vi "Main.vi"() -> ()   [LabVIEW 2020, in "ZLG_CAN.lvlib"]
doc: "This template is based off of the Queued Message Handler design pattern and the Queued Message Handler project template that ships with LabVIEW.\n\nThe main difference is that the queue is private to this module and communication between modules is performed via Broadcast and Request events.\n\nRequest events are wrapped in public API methods and are handled in the Event Handling Loop (EHL) of this VI. Any module can register for Broadcast events sent by this module. The EHL generates messages based on user interface actions.\n\nThe Message Handling Loop (MHL) processes messages generated by the EHL, or by other messages. The messages are string values, so new messages can be added easily to the Message Cases case structure in the MHL. Each message cluster can also provide an optional value for Message Data, which is a variant that can be converted to whatever message-specific data is required.\n_____\nBased on Delacor QMH Project Template 4.1.0.59."
uses:
  ZLG_CAN.lvlib
  <vilib>/Delacor/Delacor QMH/Libraries/Module Admin_class/Delacor_lib_QMH_Module Admin.lvclass
  CAN_OBJ_R.ctl
  Module Data--cluster.ctl
  <vilib>/Delacor/Delacor QMH/Libraries/Message Queue_class/Delacor_lib_QMH_Message Queue.lvclass/Delacor_lib_QMH_Message Queue.ctl
  Stop Argument--cluster.ctl
  <vilib>/Delacor/Delacor QMH/Libraries/Module Admin_class/Delacor_lib_QMH_Module Admin.lvclass/Delacor_lib_QMH_Module Admin.ctl
  Open_CAN Argument--cluster.ctl
  Init_CAN Argument--cluster.ctl
  Start_CAN Argument--cluster.ctl
  Start_CAN (Reply Payload)--cluster.ctl
  Sent_CAN Argument--cluster.ctl
  CAN_Frame.ctl
  Close_CAN Argument--cluster.ctl
  Reset_CAN Argument--cluster.ctl
  Recive_CAN Argument--cluster.ctl
  Recive_Wait Argument--cluster.ctl
  Recive_Wait (Reply Payload)--cluster.ctl
  Sent_Recive Argument--cluster.ctl
  Sent_Recive (Reply Payload)--cluster.ctl
  <vilib>/Utility/miscctls.llb/LVPointTypeDef.ctl
  CAN_OBJ_T.ctl
  <vilib>/Delacor/Delacor QMH/Libraries/Message Queue_class/Delacor_lib_QMH_Enqueue Message (Single).vi
  <vilib>/Delacor/Delacor QMH/Libraries/Module Admin_class/Delacor_lib_QMH_Get External Launch.vi
  <vilib>/Utility/error.llb/Error Cluster From Error Code.vi
  <vilib>/ErrorRing/Error Ring.xnode
  <vilib>/Delacor/Delacor QMH/Libraries/Message Queue_class/Delacor_lib_QMH_Message Queue.lvclass
  ControlCAN.dll
panel:
  out "CAN_OBJ_RN":T1[](array[typedef])
  out "CAN 通道":u32
  out "索引":u32
  out "设备类型":u32
  in  "Simulate MHL Error":bool
  in  "Simulate EHL Error":bool
  out "error out":errorcluster
  in  "Module Admin":refnum<class "Delacor_lib_QMH_Module Admin.lvclass">
  out "Status":string
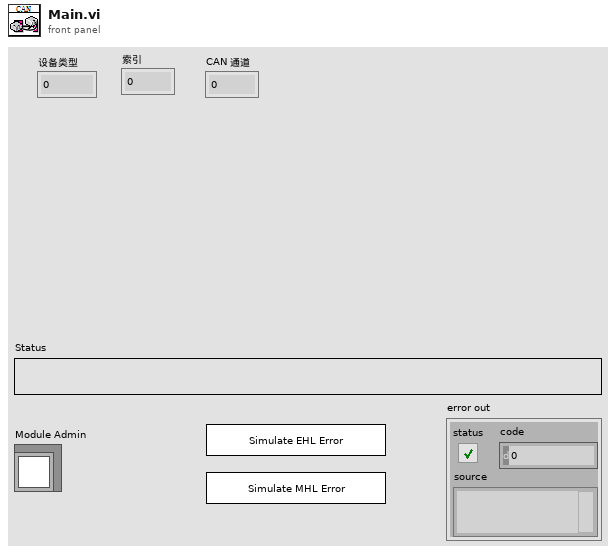
[diagram p1: front panel]
types:
  T1 = typedef "ZLG_CAN.lvlib/CAN_OBJ_R.ctl" = cluster{"ID":u32, "TimeStamp":u32, "TimeFlag":u8, "SendType":u8, "RemoteFlag":u8, "ExternFlag":u8, "DataLen":u8, "数值":u8, "数值":u8, "数值":u8, "数值":u8, "数值":u8, "数值":u8, "数值":u8, "数值":u8, "数值":u8, "数值":u8, "数值":u8}
  T2 = typedef "ZLG_CAN.lvlib/Request Events--cluster.ctl" = cluster{"Stop Module":refnum<user-event>, "Show Panel":refnum<user-event>, "Hide Panel":refnum<user-event>, "Get Module Execution Status":refnum<user-event>, "Show Diagram":refnum<user-event>, "Open_CAN":refnum<user-event>, "Init_CAN":refnum<user-event>, "Start_CAN":refnum<user-event>, "Sent_CAN":refnum<user-event>, "Close_CAN":refnum<user-event>, "Reset_CAN":refnum<user-event>, "Recive_CAN":refnum<user-event>, "Recive_Wait":refnum<user-event>, "Sent_Recive":refnum<user-event>}
  T3 = typedef "ZLG_CAN.lvlib/Module Data--cluster.ctl" = cluster{"Status":string}
  T4 = enum32{"invalid lock state", "Not Locked", "Locked (No Password)", "Password-protected"}
  T5 = typedef "ZLG_CAN.lvlib/Stop Argument--cluster.ctl" = cluster{"Origin":string, "Exit via Stop Module Req?":bool, "Wait for Module to stop?":bool}
  T6 = typedef "ZLG_CAN.lvlib/Open_CAN Argument--cluster.ctl" = cluster{"设备类型":u32, "索引":u32, "CAN 通道":u32}
  T7 = typedef "ZLG_CAN.lvlib/Init_CAN Argument--cluster.ctl" = cluster{"波特率":u32}
  T8 = typedef "ZLG_CAN.lvlib/Start_CAN Argument--cluster.ctl" = cluster{"布尔":bool, "Wait Notifier":refnum<notifier>, "wait for reply":bool}
  T9 = typedef "ZLG_CAN.lvlib/Sent_CAN Argument--cluster.ctl" = cluster{"ID":u32, "帧类型":u8, "帧格式":u8, "帧长度":u8, "CAN_FRAME":T10}
  T10 = typedef "ZLG_CAN.lvlib/CAN_Frame.ctl" = cluster{"[0]":u8, "[1]":u8, "[2]":u8, "[3]":u8, "[4]":u8, "[5]":u8, "[6]":u8, "[7]":u8}
  T11 = typedef "ZLG_CAN.lvlib/Close_CAN Argument--cluster.ctl" = cluster{"设备类型":u32, "索引":u32}
  T12 = typedef "ZLG_CAN.lvlib/Reset_CAN Argument--cluster.ctl" = cluster{"设备类型":u32, "索引":u32, "CAN 通道":u32}
  T13 = typedef "ZLG_CAN.lvlib/Recive_CAN Argument--cluster.ctl" = cluster{"布尔":bool}
  T14 = typedef "ZLG_CAN.lvlib/Recive_Wait Argument--cluster.ctl" = cluster{"Wait Notifier":refnum<notifier>, "wait for reply":bool}
  T15 = typedef "ZLG_CAN.lvlib/Sent_Recive Argument--cluster.ctl" = cluster{"ID":u32, "帧类型":u8, "帧格式":u8, "CAN_FRAME":T10, "帧长度":u8, "Wait Notifier":refnum<notifier>, "wait for reply":bool}
  T16 = typedef "LVPointTypeDef.ctl" = cluster{"Horizontal":i16, "Vertical":i16}
  T17 = enum32{"Invalid", "Standard", "Closed", "Hidden", "Minimized", "Maximized"}
  T18 = cluster{"AccCode":u32, "AccMask":u32, "Reserved":u32, "Filter":u8, "Timing0":u8, "Timing1":u8, "Mode":u8}
  T19 = typedef "ZLG_CAN.lvlib/CAN_OBJ_T.ctl" = cluster{"ID":u32, "TimeStamp":u32, "TimeFlag":u8, "SendType":u8, "RemoteFlag":u8, "ExternFlag":u8, "DataLen":u8, "CAN_Bit_0":u8, "CAN_Bit_1":u8, "CAN_Bit_2":u8, "CAN_Bit_3":u8, "CAN_Bit_4":u8, "CAN_Bit_5":u8, "CAN_Bit_6":u8, "CAN_Bit_7":u8, "CAN_Bit_8":u8, "CAN_Bit_9":u8, "CAN_Bit_10":u8}
  T20 = typedef "ZLG_CAN.lvlib/Start_CAN (Reply Payload)--cluster.ctl" = cluster{"Success":bool, "Start_CAN_error":errorcluster}
  T21 = typedef "ZLG_CAN.lvlib/Recive_Wait (Reply Payload)--cluster.ctl" = cluster{"Can_Receive":T1[], "Recive_Wait_error":errorcluster}
  T22 = typedef "ZLG_CAN.lvlib/Sent_Recive (Reply Payload)--cluster.ctl" = cluster{"Receive":T1[], "Sent_Recive_error":errorcluster}
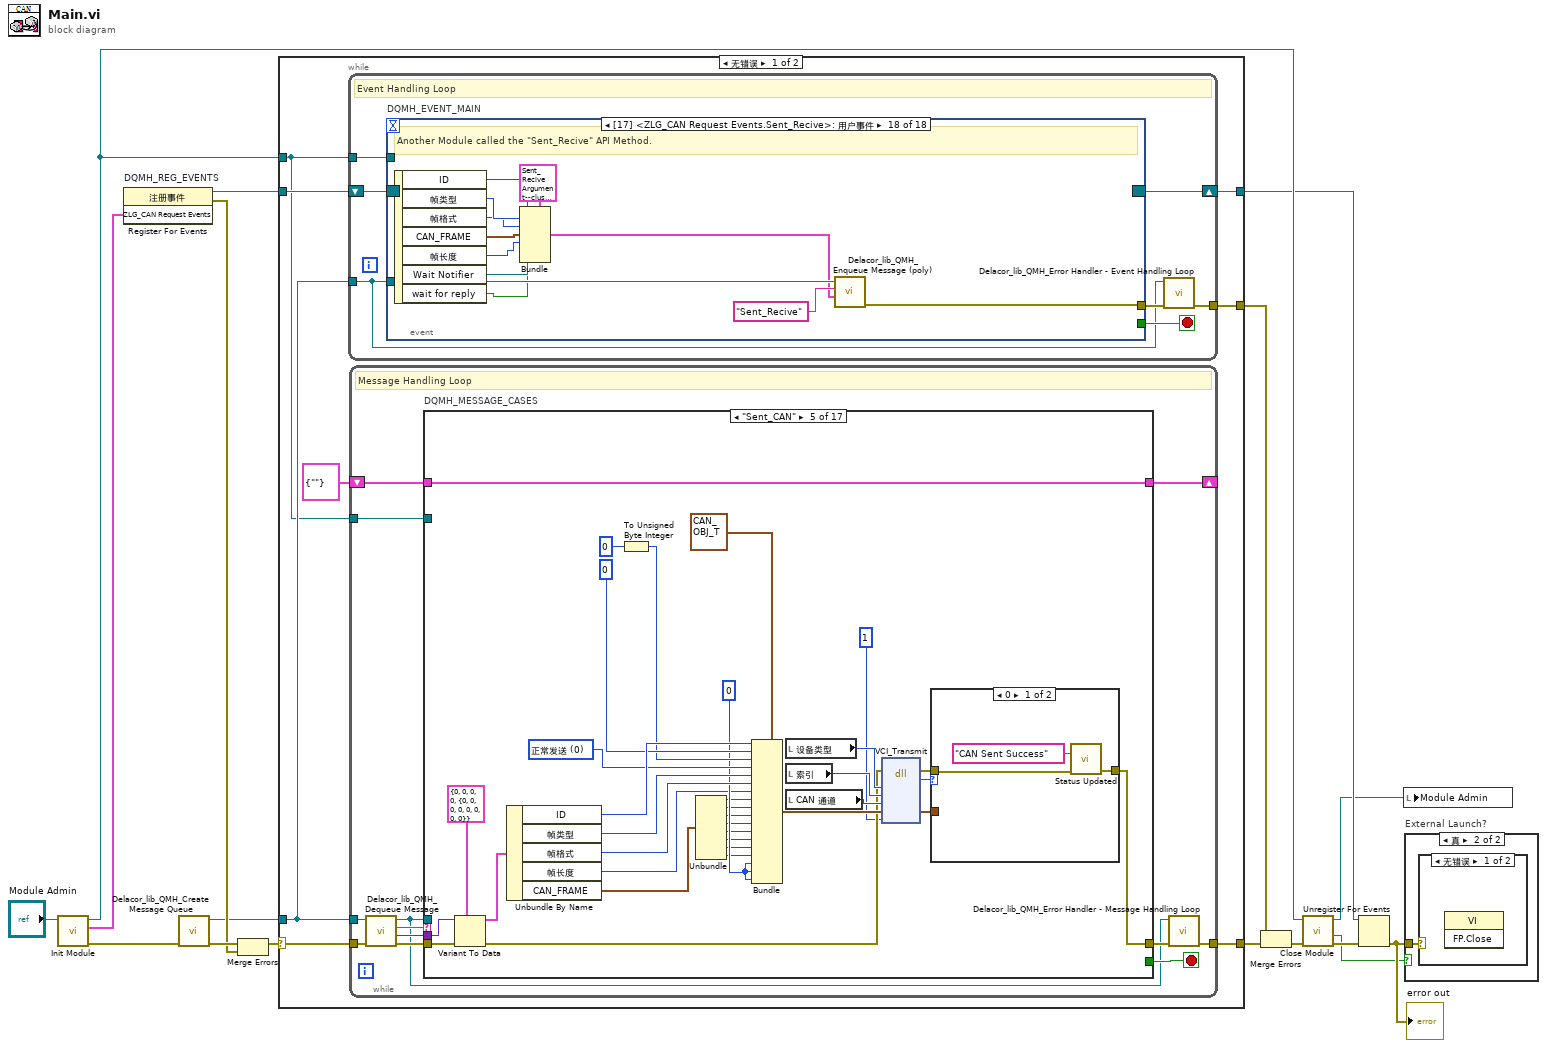
[diagram p0: block diagram]
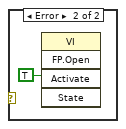
[diagram p3: hidden frame]
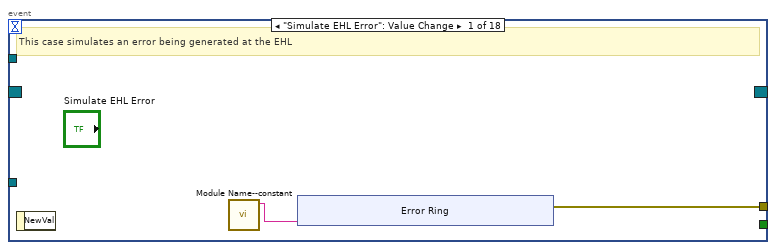
[diagram p4: hidden frame]
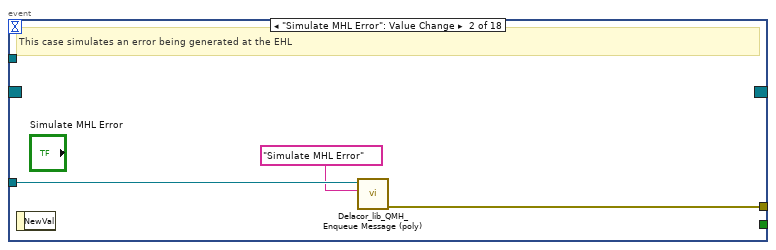
[diagram p5: hidden frame]
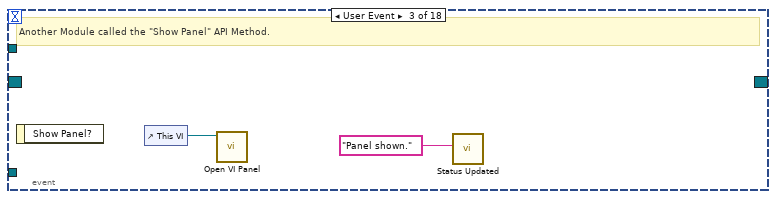
[diagram p6: hidden frame]
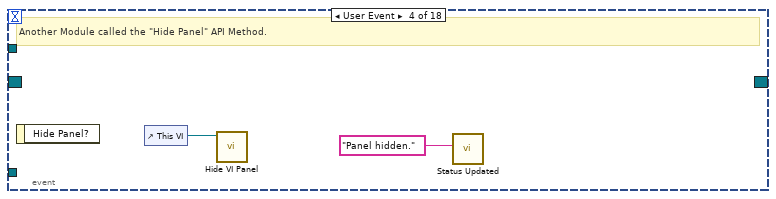
[diagram p7: hidden frame]
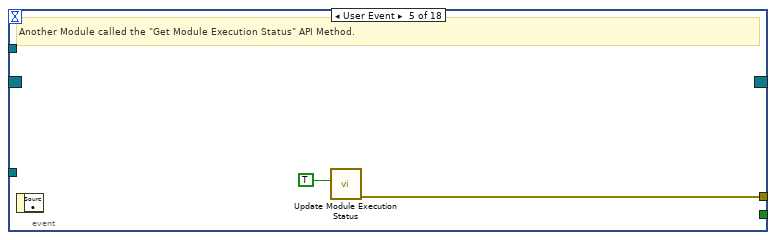
[diagram p8: hidden frame]
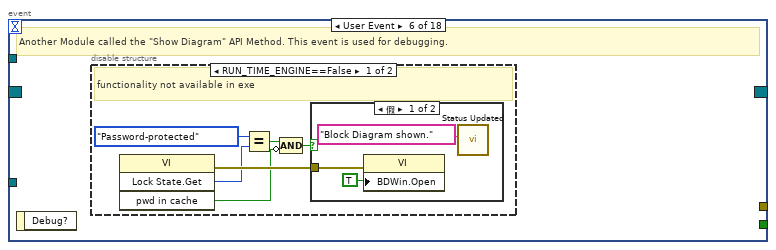
[diagram p9: hidden frame]
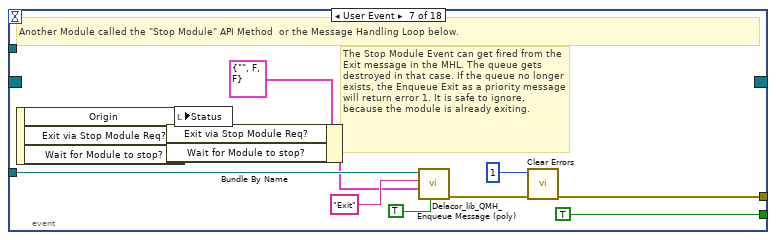
[diagram p12: hidden frame]
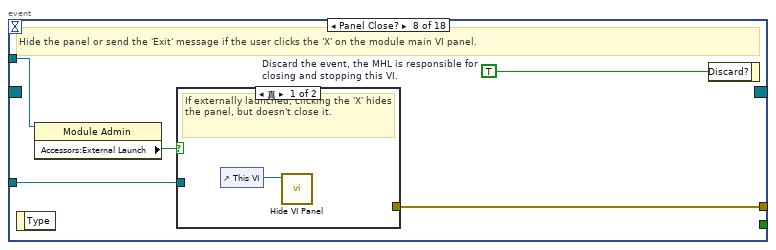
[diagram p13: hidden frame]
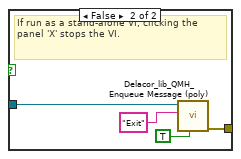
[diagram p14: hidden frame]
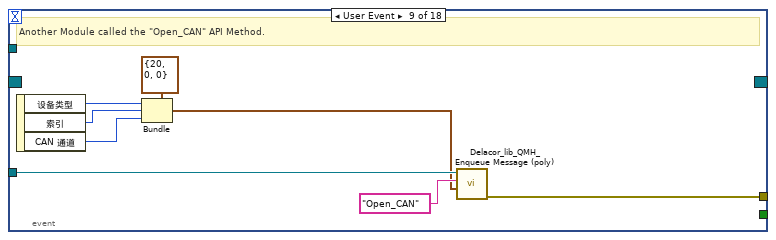
[diagram p15: hidden frame]
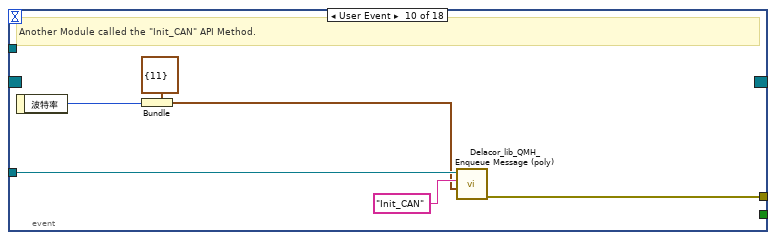
[diagram p16: hidden frame]
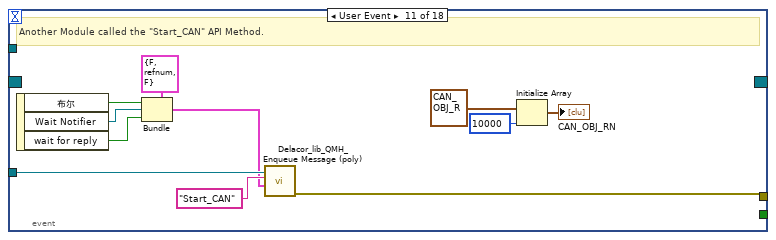
[diagram p17: hidden frame]
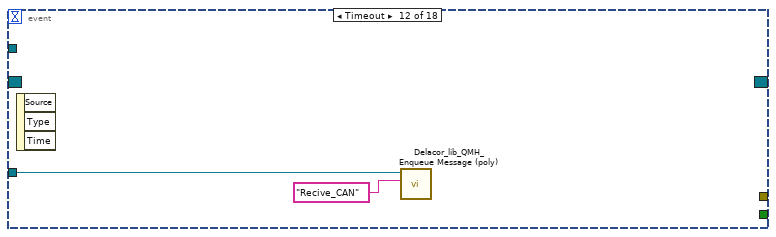
[diagram p18: hidden frame]
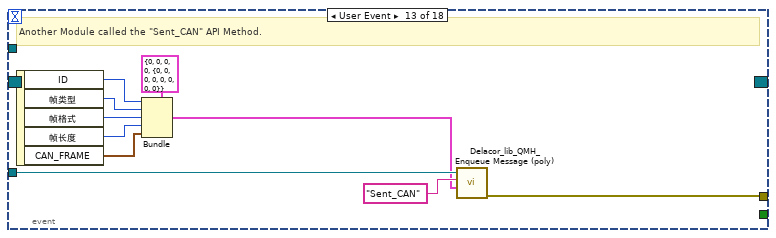
[diagram p19: hidden frame]
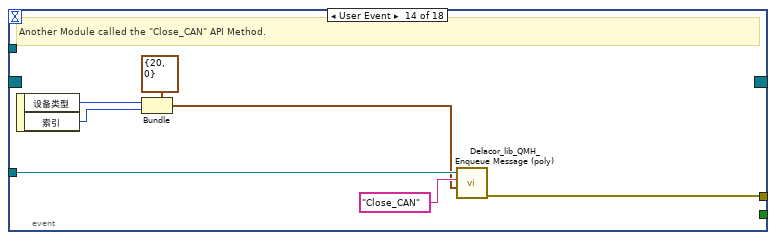
[diagram p20: hidden frame]
diagram:
  n1 = call "Init Module.vi"("Singleton Module Admin in"="Module Admin") -> ("error out"=w16:errorcluster, "ZLG_CAN Request Events"=w5:T2, "Singleton Module Admin out"=w8:refnum<class "Delacor_lib_QMH_Module Admin.lvclass">)  [unwired: 8 in]
  n2 = register-events "DQMH_REG_EVENTS"(w5) -> (reference out=w6:refnum<event-registration>, error out=w9:errorcluster)  [unwired: 2 in]
  n3 = call <vilib>:"Delacor_lib_QMH_Create Message Queue.vi"("error in"=w16) -> ("error out"=w11:errorcluster, "Message Queue"=w4:refnum<class "Delacor_lib_QMH_Message Queue.lvclass">)  [unwired: 9 in]
  n4 = Merge Errors(w11, w9) -> (w10:errorcluster)
  n5 = case shown="无错误" w10 {
    selector: w10 -> [w23 w581]
    tunnel: [w25 w581] -> w17
    tunnel: [w22 w578] -> w7
    tunnel: w6 -> [w20 w578]
    tunnel: w4 -> [w19 _]
    tunnel: [w24 _] -> w14
    tunnel: w8 -> [w18 w574]
    frame No Error {
      n6 = while {
        tunnel: w19 -> [w26]
        shift-right: [w29] -> w22
        shift-left: w20 -> [w30]
        tunnel: [w31] -> w24
        tunnel: w18 -> [w27]
        stop <- w28 stop-if-true
        # "Event Handling Loop"
        n7 = event "DQMH_EVENT_MAIN" shown="[17] <ZLG_CAN Request Events.Sent_Recive>: 用户事件" {
          selector: w30 -> [_ _ _ _ _ _ _ _ _ _ _ _ _ _ _ _ _ _]
          dyn-events: [_ _ _ _ _ _ _ _ _ _ _ _ _ _ _ _ _ _] -> w29
          timeout: _ -> [_ _ _ _ _ _ _ _ _ _ _ _ _ _ _ _ _ _]
          tunnel: [_ _ _ _ _ _ TRUE ("Discard?") _ _ _ _ _ _ _ _ _ _ _] -> w28
          tunnel: w26 -> [_ w43 _ _ _ _ w67 w74 w89 w95 w106 w107 w118 w125 w133 w139 w146 w158]
          tunnel: [w34 w44 _ _ w50 _ w70 w76 w82 w90 w101 _ w113 w119 w128 w134 w140 w147] -> w32
          tunnel: w27 -> [_ _ _ _ _ _ _ w73 _ _ _ _ _ _ _ _ _ _]
          event "Simulate EHL Error": Value Change {
            # "This case simulates an error being generated at the EHL"
            n8 = event-data() -> ()  [unwired: 1 in, 1 out]
            n9 = call "Module Name--constant.vi"() -> ("Module Name"=w33:string)  [unwired: 11 in]
            n10 = xnode "Error Ring"("参数 0"=w33) -> ("错误输出"=w34:errorcluster)
          }
          event "Simulate MHL Error": Value Change {
            # "This case simulates an error being generated at the EHL"
            n11 = event-data() -> ()  [unwired: 1 in, 1 out]
            n12 = call-poly <vilib>:"Delacor_lib_QMH_Enqueue Message (poly).vi"("Message"="Simulate MHL Error", "Message Queue in"=w43) -> ("error out"=w44:errorcluster)  [unwired: 8 in, 1 out]
          }
          event User Event {
            # "Another Module called the \"Show Panel\" API Method."
            n13 = event-data() -> ()  [unwired: 1 in, 1 out]
            n14 = control-ref of="This VI"() -> (w46:refnum<vi>)
            n15 = call "Open VI Panel.vi"("VI"=w46) -> ()  [unwired: 10 in, 1 out]
            n16 = call "Status Updated.vi"("Status"="Panel shown." ("format string")) -> ()  [unwired: 10 in, 1 out]
          }
          event User Event {
            # "Another Module called the \"Hide Panel\" API Method."
            n17 = event-data() -> ()  [unwired: 1 in, 1 out]
            n18 = control-ref of="This VI"() -> (w48:refnum<vi>)
            n19 = call "Hide VI Panel.vi"("VI"=w48) -> ()  [unwired: 10 in, 1 out]
            n20 = call "Status Updated.vi"("Status"="Panel hidden." ("format string")) -> ()  [unwired: 10 in, 1 out]
          }
          event User Event {
            # "Another Module called the \"Get Module Execution Status\" API Method."
            n21 = event-data() -> ()  [unwired: 1 in, 1 out]
            n22 = call "Update Module Execution Status.vi"("Running?"=TRUE) -> ("error out"=w50:errorcluster)  [unwired: 10 in]
          }
          event User Event {
            # "Another Module called the \"Show Diagram\" API Method. This event is used for debugging."
            n23 = event-data() -> ()  [unwired: 1 in, 1 out]
            n24 = disable-structure shown="RUN_TIME_ENGINE==False" {
              frame condition #0 (active) {
                # "functionality not available in exe"
                n25 = invoke class="VI" method="Lock State.Get"() -> (error out=w56:errorcluster, "Get Lock State"=w55:T4, "pwd in cache"=w52:bool)  [unwired: 4 in, 1 out]
                n26 = Equal?(x=T4."Password-protected", y=w55) -> (x = y?=w53:bool)
                n27 = Compound Arithmetic op=AND(w53, invert w52) -> (w51:bool)
                n28 = case "条件结构" shown="假" w51 {
                  tunnel: w56 -> [w59 _]
                  frame False {
                    n29 = property class="VI"(error in=w59, "BDWin.Open"=TRUE ("Block Diagram Window:Open")) -> ()  [unwired: 1 in, 2 out]
                    n30 = call "Status Updated.vi"("Status"="Block Diagram shown." ("format string")) -> ()  [unwired: 10 in, 1 out]
                  }
                  frame True {
                    # "Password-protected VI, and the password is not in the cache. Do not show the diagram."
                  }
                }
              }
              frame condition #1 {
              }
            }
          }
          event User Event {
            # "The Stop Module Event can get fired from the Exit message in the MHL. The queue gets destroyed in that case. If the queue no longer exists, the Enqueue Exit as a priority message will return error 1. It is safe to ignore, because the module is already exiting."
            # "Another Module called the \"Stop Module\" API Method  or the Message Handling Loop below."
            n31 = event-data() -> ("Origin"=w66:string, "Exit via Stop Module Req?"=w62:bool, "Wait for Module to stop?"=w61:bool)  [unwired: 1 in]
            n32 = Bundle By Name(cluster=T5 {"Origin"="", "Exit via Stop Module Req?"=FALSE, "Wait for Module to stop?"=FALSE} ("Stop Argument"), "Exit via Stop Module Req?"=w62, "Wait for Module to stop?"=w61) -> (w60:T5)
            n33 = local write "Status"(w66) -> ()
            n34 = call-poly <vilib>:"Delacor_lib_QMH_Enqueue Message (poly).vi"("Priority Message? (F)"=TRUE, "Message Data"=w60, "Message"="Exit", "Message Queue in"=w67) -> ("error out"=w71:errorcluster)  [unwired: 6 in, 1 out]
            n35 = call <vilib>:"Clear Errors.vi"("error in (no error)"=w71, "specific error code to clear (0: all)"=1) -> ("error out"=w70:errorcluster)  [unwired: 4 in, 1 out]
          }
          event Panel Close? {
            w75 = TRUE  # Discard the event, the MHL is responsible for closing and stopping this VI.
            # "Hide the panel or send the 'Exit' message if the user clicks the 'X' on the module main VI panel."
            n36 = event-data() -> ()  [unwired: 1 in, 1 out]
            n37 = property class="Module Admin"(reference=w73) -> ("Accessors:External Launch"=w72:bool)  [unwired: 1 in, 2 out]
            n38 = case "条件结构" shown="真" w72 {
              tunnel: w74 -> [_ w80]
              tunnel: [_ w81] -> w76
              frame True {
                # "If externally launched, clicking the 'X' hides the panel, but doesn't close it."
                n39 = control-ref of="This VI"() -> (w77:refnum<vi>)
                n40 = call "Hide VI Panel.vi"("VI"=w77) -> ()  [unwired: 10 in, 1 out]
              }
              frame False {
                # "If run as a stand-alone VI, clicking the panel 'X' stops the VI."
                n41 = call-poly <vilib>:"Delacor_lib_QMH_Enqueue Message (poly).vi"("Priority Message? (F)"=TRUE, "Message"="Exit", "Message Queue in"=w80) -> ("error out"=w81:errorcluster)  [unwired: 7 in, 1 out]
              }
            }
            n42 = event-data("Discard?"=w75) -> ()  [unwired: 1 in, 1 out]
          }
          event User Event {
            # "Another Module called the \"Open_CAN\" API Method."
            n43 = event-data() -> ("设备类型"=w85:u32, "索引"=w84:u32, "CAN 通道"=w83:u32)  [unwired: 1 in]
            n44 = Bundle(cluster=T6 {"设备类型"=20, "索引"=0, "CAN 通道"=0} ("Open_CAN Argument"), "设备类型"=w85, "索引"=w84, "CAN 通道"=w83) -> (w86:T6)
            n45 = call-poly <vilib>:"Delacor_lib_QMH_Enqueue Message (poly).vi"("Message Data"=w86, "Message"="Open_CAN", "Message Queue in"=w89) -> ("error out"=w82:errorcluster)  [unwired: 7 in, 1 out]
          }
          event User Event {
            # "Another Module called the \"Init_CAN\" API Method."
            n46 = event-data() -> ("波特率"=w91:u32)  [unwired: 1 in]
            n47 = Bundle(cluster=T7 {"波特率"=11} ("Init_CAN Argument"), "波特率"=w91) -> (w92:T7)
            n48 = call-poly <vilib>:"Delacor_lib_QMH_Enqueue Message (poly).vi"("Message Data"=w92, "Message"="Init_CAN", "Message Queue in"=w95) -> ("error out"=w90:errorcluster)  [unwired: 7 in, 1 out]
          }
          event User Event {
            # "Another Module called the \"Start_CAN\" API Method."
            n49 = event-data() -> ("布尔"=w102:bool, "Wait Notifier"=w100:refnum<notifier>, "wait for reply"=w99:bool)  [unwired: 1 in]
            n50 = Bundle(cluster=T8 {"布尔"=FALSE, "Wait Notifier"=refnum, "wait for reply"=FALSE} ("Start_CAN Argument"), "布尔"=w102, "Wait Notifier"=w100, "wait for reply"=w99) -> (w103:T8)
            n51 = call-poly <vilib>:"Delacor_lib_QMH_Enqueue Message (poly).vi"("Message Data"=w103, "Message"="Start_CAN", "Message Queue in"=w106) -> ("error out"=w101:errorcluster)  [unwired: 7 in, 1 out]
            n52 = Initialize Array(T1 {"ID"=0, "TimeStamp"=0, "TimeFlag"=0, "SendType"=1, "RemoteFlag"=0, "ExternFlag"=0, "DataLen"=8, "数值"=0, "数值"=0, "数值"=0, "数值"=0, "数值"=0, "数值"=0, "数值"=0, "数值"=0, "数值"=0, "数值"=0, "数值"=0} ("CAN_OBJ_R"), 10000 ("维数大小")) -> (→"CAN_OBJ_RN":T1[])
          }
          event Timeout {
            n53 = event-data() -> ()  [unwired: 1 in, 3 out]
            n54 = call-poly <vilib>:"Delacor_lib_QMH_Enqueue Message (poly).vi"("Message"="Recive_CAN", "Message Queue in"=w107) -> ()  [unwired: 8 in, 2 out]
          }
          event User Event {
            # "Another Module called the \"Sent_CAN\" API Method."
            n55 = event-data() -> ("ID"=w114:u32, "帧类型"=w112:u8, "帧格式"=w111:u8, "帧长度"=w110:u8, "CAN_FRAME"=w109:T10)  [unwired: 1 in]
            n56 = Bundle(cluster=T9 {"ID"=0, "帧类型"=0, "帧格式"=0, "帧长度"=0, "CAN_FRAME"={"[0]"=0, "[1]"=0, "[2]"=0, "[3]"=0, "[4]"=0, "[5]"=0, "[6]"=0, "[7]"=0}} ("Sent_CAN Argument"), "ID"=w114, "帧类型"=w112, "帧格式"=w111, "帧长度"=w110, "CAN_FRAME"=w109) -> (w115:T9)
            n57 = call-poly <vilib>:"Delacor_lib_QMH_Enqueue Message (poly).vi"("Message Data"=w115, "Message"="Sent_CAN", "Message Queue in"=w118) -> ("error out"=w113:errorcluster)  [unwired: 7 in, 1 out]
          }
          event User Event {
            # "Another Module called the \"Close_CAN\" API Method."
            n58 = event-data() -> ("设备类型"=w121:u32, "索引"=w120:u32)  [unwired: 1 in]
            n59 = Bundle(cluster=T11 {"设备类型"=20, "索引"=0} ("Close_CAN Argument"), "设备类型"=w121, "索引"=w120) -> (w122:T11)
            n60 = call-poly <vilib>:"Delacor_lib_QMH_Enqueue Message (poly).vi"("Message Data"=w122, "Message"="Close_CAN", "Message Queue in"=w125) -> ("error out"=w119:errorcluster)  [unwired: 7 in, 1 out]
          }
          event User Event {
            # "Another Module called the \"Reset_CAN\" API Method."
            n61 = event-data() -> ("设备类型"=w129:u32, "索引"=w127:u32, "CAN 通道"=w126:u32)  [unwired: 1 in]
            n62 = Bundle(cluster=T12 {"设备类型"=20, "索引"=0, "CAN 通道"=0} ("Reset_CAN Argument"), "设备类型"=w129, "索引"=w127, "CAN 通道"=w126) -> (w130:T12)
            n63 = call-poly <vilib>:"Delacor_lib_QMH_Enqueue Message (poly).vi"("Message Data"=w130, "Message"="Reset_CAN", "Message Queue in"=w133) -> ("error out"=w128:errorcluster)  [unwired: 7 in, 1 out]
          }
          event User Event {
            # "Another Module called the \"Recive_CAN\" API Method."
            n64 = event-data() -> ("布尔"=w135:bool)  [unwired: 1 in]
            n65 = Bundle(cluster=T13 {"布尔"=FALSE} ("Recive_CAN Argument"), "布尔"=w135) -> (w136:T13)
            n66 = call-poly <vilib>:"Delacor_lib_QMH_Enqueue Message (poly).vi"("Message Data"=w136, "Message"="Recive_CAN", "Message Queue in"=w139) -> ("error out"=w134:errorcluster)  [unwired: 7 in, 1 out]
          }
          event User Event {
            # "Another Module called the \"Recive_Wait\" API Method."
            n67 = event-data() -> ("Wait Notifier"=w142:refnum<notifier>, "wait for reply"=w141:bool)  [unwired: 1 in]
            n68 = Bundle(cluster=T14 {"Wait Notifier"=refnum, "wait for reply"=FALSE} ("Recive_Wait Argument"), "Wait Notifier"=w142, "wait for reply"=w141) -> (w143:T14)
            n69 = call-poly <vilib>:"Delacor_lib_QMH_Enqueue Message (poly).vi"("Message Data"=w143, "Message"="Recive_Wait", "Message Queue in"=w146) -> ("error out"=w140:errorcluster)  [unwired: 7 in, 1 out]
          }
          event User Event {
            # "Another Module called the \"Sent_Recive\" API Method."
            n70 = event-data() -> ("ID"=w154:u32, "帧类型"=w153:u8, "帧格式"=w152:u8, "CAN_FRAME"=w151:T10, "帧长度"=w150:u8, "Wait Notifier"=w149:refnum<notifier>, "wait for reply"=w148:bool)  [unwired: 1 in]
            n71 = Bundle(cluster=T15 {"ID"=0, "帧类型"=0, "帧格式"=0, "CAN_FRAME"={"[0]"=0, "[1]"=0, "[2]"=0, "[3]"=0, "[4]"=0, "[5]"=0, "[6]"=0, "[7]"=0}, "帧长度"=0, "Wait Notifier"=refnum, "wait for reply"=FALSE} ("Sent_Recive Argument"), "ID"=w154, "帧类型"=w153, "帧格式"=w152, "CAN_FRAME"=w151, "帧长度"=w150, "Wait Notifier"=w149, "wait for reply"=w148) -> (w155:T15)
            n72 = call-poly <vilib>:"Delacor_lib_QMH_Enqueue Message (poly).vi"("Message Data"=w155, "Message"="Sent_Recive", "Message Queue in"=w158) -> ("error out"=w147:errorcluster)  [unwired: 7 in, 1 out]
          }
        }
        n73 = call-dynamic "Delacor_lib_QMH_Error Handler - Event Handling Loop.vi"("error in"=w32, "Message Queue in"=w26) -> ("dup error in"=w31:errorcluster)  [unwired: 8 in, 1 out]
      }
      n74 = while {
        tunnel: w19 -> [w161]
        shift-right: [w165] -> _
        shift-left: T3 {"Status"=""} ("Data Cluster") -> [w166]
        tunnel: w23 -> [w169]
        tunnel: [w167] -> w25
        tunnel: w18 -> [w159]
        stop <- w164 stop-if-true
        # "Message Handling Loop"
        n75 = call-dynamic "Delacor_lib_QMH_Dequeue Message.vi"("error in"=w169, "Message Queue in"=w161) -> ("error out"=w168:errorcluster, "Message Data"=w162:variant, "Message"=w163:string, "Message Queue out"=w160:refnum<class "Delacor_lib_QMH_Message Queue.lvclass">)  [unwired: 6 in]
        n76 = case "DQMH_MESSAGE_CASES" shown="\"Sent_CAN\"" w163 {
          selector: w163 -> [_ _ _ _ _ _ _ _ _ _ _ _ _ _ _ _ w561]
          tunnel: w160 -> [_ _ _ _ _ _ _ _ _ _ _ _ _ _ w531 w553 _]
          tunnel: w168 -> [w188 w192 w205 w231 w303 w325 w343 w367 w385 w424 w487 w514 w516 w521 w538 w559 w563]
          tunnel: [w186 w192 w195 w212 w271 w317 w337 w359 w378 w412 w482 w513 w516 w520 w534 w556 w564] -> w170
          tunnel: w166 -> [w177 w191 w204 w230 w302 w324 w342 w366 w384 w423 w486 w512 w515 w518 w533 w552 w562]
          tunnel: [w176 w191 w204 w230 w302 w324 w342 w366 w384 w423 w486 w512 w515 w518 w533 w552 w562] -> w165
          tunnel: [_ _ _ _ _ _ _ _ _ _ _ _ _ _ _ w551 _] -> w164
          tunnel: w162 -> [_ _ w203 w229 w301 w323 w341 w365 w383 w422 w485 _ _ _ w532 w550 _]
          tunnel: w159 -> [w178 _ _ _ _ _ _ _ _ _ _ _ _ _ w530 w545 _]
          frame "Initialize" {
            w171 = "Initial Message" ("Initial Message")
            # "#CodeNeeded - Initialize the appearance of the front panel."
            # "#CodeNeeded - Initialize your state data here."
            # "Initialize - Any operation that needs to be done before the module can receive messages. Synchronize Caller Events.vi will inform Start Module.vi that the module has launched and is ready to receive messages. Module Did Init.vi will broadcast that the module initialized."
            n77 = call "Synchronize Caller Events.vi"("error in (no error)"=w188, "Singleton Module Admin in"=w178) -> ("error out"=w187:errorcluster, "Singleton Module Admin out"=w173:refnum<class "Delacor_lib_QMH_Module Admin.lvclass">)  [unwired: 8 in]
            n78 = property class="Module Admin"(reference=w173) -> ("Accessors:External Launch"=w182:bool)  [unwired: 1 in, 2 out]
            n79 = Select(t=T17."Hidden" ("State"), s=w182, f=T17."Standard" ("State")) -> (s? t:f=w179:T17)
            n80 = call "Module Name--constant.vi"() -> ("Module Name"=w185:string)  [unwired: 11 in]
            n81 = property class="VI"("Front Panel.Title"=w185) -> (reference out=w184:refnum<vi>, error out=w190:errorcluster)  [unwired: 2 in]
            n82 = call "Module Name--constant.vi"() -> ("Module Name"=w174:string)  [unwired: 11 in]
            n83 = invoke class="VI" method="FP.Open"(reference=w184, error in=w190, "State"=w179) -> (reference out=w183:refnum<vi>, error out=w189:errorcluster)  [unwired: 2 in, 3 out]
            n84 = Bundle By Name(cluster=w177, "Status"=w171) -> (w176:T3)
            n85 = call "Module Did Init.vi"("error in (no error)"=w187, "Initialized?"=TRUE, "Origin"=w174) -> ("error out"=w186:errorcluster)  [unwired: 8 in]
            n86 = invoke class="VI" method="FP.Center"(reference=w183, error in=w189) -> ()  [unwired: 1 in, 3 out]
            n87 = property on="Pane" class="Pane"("Origin"=T16 {"Horizontal"=0, "Vertical"=0}) -> ()  [unwired: 2 in, 2 out]
            "Status" <- w171
          }
          frame "--- Module Specific ---" {
            # "Separator -- The following cases handle messages specific to this Module."
          }
          frame "Open_CAN" {
            n88 = Variant To Data(error in=w205, type=T6 {"设备类型"=20, "索引"=0, "CAN 通道"=0} ("Open_CAN Argument"), Variant=w203) -> (data=w201:T6, error out=w198:errorcluster)
            n89 = Unbundle By Name(w201) -> ("设备类型"=w200:u32, "索引"=w193:u32, "CAN 通道"=→"CAN 通道":u32)
            "设备类型" <- w200
            "索引" <- w193
            n90 = dll-call lib="PTH2labs CUsers\n终极BOSS\tDocumentsCEPSLV300-1老性能试验台\tLibrariesZLG_CANControlCAN.dll" fn="VCI_OpenDevice"(error in=w198, "DevType"=w200, "DevIndex"=w193, "Reserved"=u32 0) -> (error out=w196:errorcluster, "返回类型"=w197:u32)  [unwired: 5 in, 1 out]
            n91 = case shown="0, 默认" w197 {
              tunnel: w196 -> [w207 w210]
              tunnel: [w206 w209] -> w195
              frame 0, Default {
                n92 = call "Status Updated.vi"("error in (no error)"=w207, "Status"="CAN Open Faild" ("format string")) -> ("error out"=w206:errorcluster)  [unwired: 9 in]
              }
              frame 1 {
                n93 = call "Status Updated.vi"("error in (no error)"=w210, "Status"="CAN Open Success" ("format string")) -> ("error out"=w209:errorcluster)  [unwired: 9 in]
              }
            }
          }
          frame "Init_CAN" {
            w221 = u32 0 ("Reserved")
            n94 = Variant To Data(error in=w231, type=T7 {"波特率"=11} ("Init_CAN Argument"), Variant=w229) -> (data=w227:T7, error out=w215:errorcluster)
            n95 = Unbundle By Name(w227) -> ("波特率"=w220:u32)
            n96 = case shown="14" w220 {
              tunnel: [u8 191 ("BTR0") 49 24 135 9 131 4 3 250 1 128 0 128 0 0 1] -> w226
              tunnel: [u8 255 ("BTR1") 28 28 255 28 255 28 28 129 28 250 28 182 22 20 1] -> w225
              frame 0 {
              }
              frame 1 {
              }
              frame 2 {
              }
              frame 3 {
              }
              frame 4 {
              }
              frame 5 {
              }
              frame 6 {
              }
              frame 7 {
              }
              frame 8 {
              }
              frame 9 {
              }
              frame 10 {
              }
              frame 11 {
              }
              frame 12 {
              }
              frame 13 {
              }
              frame 14 {
              }
              frame 15, Default {
              }
            }
            n97 = local read "设备类型"() -> (w216:u32)
            n98 = local read "索引"() -> (w217:u32)
            n99 = local read "CAN 通道"() -> (w218:u32)
            n100 = Bundle(cluster=T18 {"AccCode"=0, "AccMask"=4294967295, "Reserved"=0, "Filter"=0, "Timing0"=3, "Timing1"=28, "Mode"=0} ("VCI_INIT_CONFIG"), "AccCode"=u32 0 ("验收码"), "AccMask"=u32 4294967295 ("屏蔽码"), "Reserved"=w221, "Filter"=w221, "Timing0"=w226, "Timing1"=w225, "Mode"=w221) -> (w219:T18)
            n101 = dll-call lib="PTH2labs CUsers\n终极BOSS\tDocumentsCEPSLV300-1老性能试验台\tLibrariesZLG_CANControlCAN.dll" fn="VCI_InitCAN"(error in=w215, "DeviceType"=w216, "DeviceInd"=w217, "CANInd"=w218, "pInitConfig"=w219) -> (error out=w213:errorcluster, "返回类型"=w214:u32)  [unwired: 6 in, 1 out]
            n102 = case shown="1" w214 {
              tunnel: w213 -> [w233 w236]
              tunnel: [w232 w235] -> w212
              frame 0, Default {
                n103 = call "Status Updated.vi"("error in (no error)"=w233, "Status"="CAN Init Faild" ("format string")) -> ("error out"=w232:errorcluster)  [unwired: 9 in]
              }
              frame 1 {
                n104 = call "Status Updated.vi"("error in (no error)"=w236, "Status"="CAN Init Success" ("format string")) -> ("error out"=w235:errorcluster)  [unwired: 9 in]
              }
            }
          }
          frame "Sent_CAN" {
            w290 = u8 0 ("CAN_Bit_7")
            w293 = u8 0 items=["正常发送", "单次发送", "自发自收", "单次自发自收"] ("发送类型")
            n105 = Variant To Data(error in=w303, type=T9 {"ID"=0, "帧类型"=0, "帧格式"=0, "帧长度"=0, "CAN_FRAME"={"[0]"=0, "[1]"=0, "[2]"=0, "[3]"=0, "[4]"=0, "[5]"=0, "[6]"=0, "[7]"=0}} ("Sent_CAN Argument"), Variant=w301) -> (data=w299:T9, error out=w275:errorcluster)
            n106 = Unbundle By Name(w299) -> ("ID"=w297:u32, "帧类型"=w292:u8, "帧格式"=w291:u8, "帧长度"=w287:u8, "CAN_FRAME"=w288:T10)
            n107 = To Unsigned Byte Integer(number=u32 0) -> (unsigned 8bit integer=w294:u8)
            n108 = Unbundle(w288) -> ("[0]"=w286:u8, "[1]"=w285:u8, "[2]"=w284:u8, "[3]"=w283:u8, "[4]"=w282:u8, "[5]"=w281:u8, "[6]"=w280:u8, "[7]"=w279:u8)
            n109 = Bundle(cluster=T19 {"ID"=0, "TimeStamp"=0, "TimeFlag"=0, "SendType"=0, "RemoteFlag"=0, "ExternFlag"=0, "DataLen"=0, "CAN_Bit_0"=0, "CAN_Bit_1"=0, "CAN_Bit_2"=0, "CAN_Bit_3"=0, "CAN_Bit_4"=0, "CAN_Bit_5"=0, "CAN_Bit_6"=0, "CAN_Bit_7"=0, "CAN_Bit_8"=0, "CAN_Bit_9"=0, "CAN_Bit_10"=0} ("VCI_CAN_OBJ_T"), "ID"=w297, "TimeStamp"=u32 0, "TimeFlag"=w294, "SendType"=w293, "RemoteFlag"=w292, "ExternFlag"=w291, "DataLen"=w287, "CAN_Bit_0"=w286, "CAN_Bit_1"=w285, "CAN_Bit_2"=w284, "CAN_Bit_3"=w283, "CAN_Bit_4"=w282, "CAN_Bit_5"=w281, "CAN_Bit_6"=w280, "CAN_Bit_7"=w279, "CAN_Bit_8"=w290, "CAN_Bit_9"=w290, "CAN_Bit_10"=w290) -> (w289:T19)
            n110 = local read "设备类型"() -> (w276:u32)
            n111 = local read "索引"() -> (w278:u32)
            n112 = local read "CAN 通道"() -> (w277:u32)
            n113 = dll-call lib="PTH2labs CUsers\n终极BOSS\tDocumentsCEPSLV300-1老性能试验台\tLibrariesZLG_CANControlCAN.dll" fn="VCI_Transmit"(error in=w275, "DeviceType"=w276, "DeviceInd"=w278, "CANInd"=w277, "pSend"=w289, "Len"=u32 1) -> (error out=w272:errorcluster, "return type"=w273:u32, "pSend"=w270:T19)  [unwired: 6 in, 1 out]
            n114 = case shown="0" w273 {
              tunnel: w272 -> [w305 w314]
              tunnel: [w304 w312] -> w271
              tunnel: w270 -> [_ w310]
              frame 0 {
                n115 = call "Status Updated.vi"("error in (no error)"=w305, "Status"="CAN Sent Success" ("format string")) -> ("error out"=w304:errorcluster)  [unwired: 9 in]
              }
              frame 1, Default {
                n116 = call "Status Updated.vi"("error in (no error)"=w314, "Status"="CAN Sent Failed" ("format string")) -> ("error out"=w313:errorcluster)  [unwired: 9 in]
                n117 = Build Array(w310) -> (w309:T19[])
                n118 = call "CAN_Recive.vi"("error in (no error)"=w313, "T?R"=TRUE, "CAN_OBJ_RN"=w309, "NUM"=u16 1) -> ("error out"=w312:errorcluster)  [unwired: 7 in]
              }
            }
          }
          frame "Close_CAN" {
            n119 = Variant To Data(error in=w325, type=T11 {"设备类型"=20, "索引"=0} ("Close_CAN Argument"), Variant=w323) -> (data=w321:T11, error out=w318:errorcluster)
            n120 = Unbundle By Name(w321) -> ("设备类型"=w320:u32)
            n121 = dll-call lib="PTH2labs CUsers\n终极BOSS\tDocumentsCEPSLV300-1老性能试验台\tLibrariesZLG_CANControlCAN.dll" fn="VCI_CloseDevice"(error in=w318, "DeviceType"=w320, "DeviceInd"=u32 0) -> (error out=w319:errorcluster, "返回类型"=w316:u32)  [unwired: 4 in, 1 out]
            n122 = case shown="1" w316 {
              tunnel: w319 -> [w327 w330]
              tunnel: [w326 w329] -> w317
              frame 0, Default {
                n123 = call "Status Updated.vi"("error in (no error)"=w327, "Status"="CAN Close Faild" ("format string")) -> ("error out"=w326:errorcluster)  [unwired: 9 in]
              }
              frame 1 {
                n124 = call "Status Updated.vi"("error in (no error)"=w330, "Status"="CAN Close Success" ("format string")) -> ("error out"=w329:errorcluster)  [unwired: 9 in]
              }
            }
          }
          frame "Reset_CAN" {
            n125 = Variant To Data(error in=w343, type=T12 {"设备类型"=20, "索引"=0, "CAN 通道"=0} ("Reset_CAN Argument"), Variant=w341) -> (data=w339:T12, error out=w338:errorcluster)
            n126 = Unbundle By Name(w339) -> ("设备类型"=w334:u32, "索引"=w333:u32, "CAN 通道"=w332:u32)
            n127 = dll-call lib="PTH2labs CUsers\n终极BOSS\tDocumentsCEPSLV300-1老性能试验台\tLibrariesZLG_CANControlCAN.dll" fn="VCI_ResetCAN"(error in=w338, "DeviceType"=w334, "DeviceInd"=w333, "CANInd"=w332) -> (error out=w335:errorcluster, "返回类型"=w336:u32)  [unwired: 5 in, 1 out]
            n128 = case shown="1" w336 {
              tunnel: w335 -> [w344 w348]
              tunnel: [w345 w347] -> w337
              frame 0, Default {
                n129 = call "Status Updated.vi"("error in (no error)"=w344, "Status"="CAN Reset Faild" ("format string")) -> ("error out"=w345:errorcluster)  [unwired: 9 in]
              }
              frame 1 {
                n130 = call "Status Updated.vi"("error in (no error)"=w348, "Status"="CAN Reset Success" ("format string")) -> ("error out"=w347:errorcluster)  [unwired: 9 in]
              }
            }
          }
          frame "Start_CAN" {
            n131 = Variant To Data(error in=w367, type=T8 {"布尔"=FALSE, "Wait Notifier"=refnum, "wait for reply"=FALSE} ("Start_CAN Argument"), Variant=w365) -> (data=w363:T8, error out=w353:errorcluster)
            n132 = Unbundle By Name(w363) -> ("Wait Notifier"=w362:refnum<notifier>, "wait for reply"=w352:bool)
            n133 = local read "CAN 通道"() -> (w357:u32)
            n134 = local read "设备类型"() -> (w358:u32)
            n135 = local read "索引"() -> (w354:u32)
            n136 = dll-call lib="PTH2labs CUsers\n终极BOSS\tDocumentsCEPSLV300-1老性能试验台\tLibrariesZLG_CANControlCAN.dll" fn="VCI_StartCAN"(error in=w353, "DeviceType"=w358, "DeviceInd"=w354, "CANInd"=w357) -> (error out=w356:errorcluster, "返回类型"=w355:u32)  [unwired: 5 in, 1 out]
            n137 = case shown="1" w355 {
              tunnel: w356 -> [w370 w374]
              tunnel: [w369 w373] -> w350
              tunnel: [FALSE TRUE] -> w351
              frame 0, Default {
                n138 = call "Status Updated.vi"("error in (no error)"=w370, "Status"="CAN Start Faild" ("format string")) -> ("error out"=w369:errorcluster)  [unwired: 9 in]
              }
              frame 1 {
                n139 = call "Status Updated.vi"("error in (no error)"=w374, "Status"="CAN Start Success" ("format string")) -> ("error out"=w373:errorcluster)  [unwired: 9 in]
              }
            }
            n140 = Bundle By Name(cluster=T20 {"Success"=FALSE, "Start_CAN_error"={"status"=FALSE, "code"=0, "source"=""}} ("Start_CAN (Reply Payload)"), "Success"=w351, "Start_CAN_error"=w350) -> (w361:T20)
            n141 = case shown="真" w352 {
              tunnel: w362 -> [_ w377]
              tunnel: w361 -> [_ w376]
              frame False {
              }
              frame True {
                n142 = Send Notification(notification=w376, notifier=w377) -> ()  [unwired: 1 in, 2 out]
              }
            }
            n143 = Merge Errors(w353, w350) -> (w359:errorcluster)
          }
          frame "Recive_CAN" {
            n144 = Variant To Data(error in=w385, type=T13 {"布尔"=FALSE} ("Recive_CAN Argument"), Variant=w383) -> (data=w381:T13, error out=w379:errorcluster)
            n145 = Unbundle By Name(w381) -> ("布尔"=w380:bool)
            n146 = case shown="真" w380 {
              tunnel: w379 -> [w386 w388]
              tunnel: [w386 w387] -> w378
              frame False {
              }
              frame True {
                n147 = local read "CAN 通道"() -> (w391:u32)
                n148 = local read "设备类型"() -> (w393:u32)
                n149 = local read "索引"() -> (w392:u32)
                n150 = dll-call lib="PTH2labs CUsers\n终极BOSS\tDocumentsCEPSLV300-1老性能试验台\tLibrariesZLG_CANControlCAN.dll" fn="VCI_GetReceiveNum"(error in=w388, "DeviceType"=w393, "DeviceInd"=w392, "CANInd"=w391) -> (error out=w390:errorcluster, "return type"=w389:u32)  [unwired: 5 in, 1 out]
                n151 = case shown="1, 默认" w389 {
                  selector: w389 -> [_ w395]
                  tunnel: w390 -> [w394 w398]
                  tunnel: w393 -> [_ w405]
                  tunnel: w392 -> [_ w404]
                  tunnel: w391 -> [_ w403]
                  tunnel: [w394 w396] -> w387
                  frame 0 {
                  }
                  frame 1, Default {
                    n152 = local read "CAN_OBJ_RN"() -> (w402:T1[])
                    n153 = dll-call lib="PTH2labs CUsers\n终极BOSS\tDocumentsCEPSLV300-1老性能试验台\tLibrariesZLG_CANControlCAN.dll" fn="VCI_Receive"(error in=w398, "DeviceType"=w405, "DeviceInd"=w404, "CANInd"=w403, "pReceive"=w402, "Len"=w395, "WaitTime"=100) -> (error out=w397:errorcluster, "return type"=w400:u32, "pReceive"=w399:T1[])  [unwired: 7 in, 1 out]
                    n154 = case shown="1" w400 {
                      tunnel: w399 -> [_ w409]
                      tunnel: w397 -> [w406 w411]
                      tunnel: [w406 w410] -> w396
                      tunnel: w395 -> [_ w408]
                      frame 0, Default {
                      }
                      frame 1 {
                        n155 = call "CAN_Recive.vi"("error in (no error)"=w411, "T?R"=FALSE, "CAN_OBJ_RN"=w409, "NUM"=w408) -> ("error out"=w410:errorcluster)  [unwired: 7 in]
                      }
                    }
                  }
                }
              }
            }
          }
          frame "Recive_Wait" {
            n156 = Variant To Data(error in=w424, type=T14 {"Wait Notifier"=refnum, "wait for reply"=FALSE} ("Recive_Wait Argument"), Variant=w422) -> (data=w414:T14, error out=w415:errorcluster)
            n157 = local read "CAN 通道"() -> (w418:u32)
            n158 = local read "设备类型"() -> (w416:u32)
            n159 = local read "索引"() -> (w417:u32)
            n160 = dll-call lib="PTH2labs CUsers\n终极BOSS\tDocumentsCEPSLV300-1老性能试验台\tLibrariesZLG_CANControlCAN.dll" fn="VCI_GetReceiveNum"(error in=w415, "DeviceType"=w416, "DeviceInd"=w417, "CANInd"=w418) -> (error out=w419:errorcluster, "return type"=w420:u32)  [unwired: 5 in, 1 out]
            n161 = case shown="1, 默认" w420 {
              selector: w420 -> [w430 _]
              tunnel: w419 -> [w431 w442]
              tunnel: w416 -> [w436 _]
              tunnel: w417 -> [w435 _]
              tunnel: w418 -> [w434 _]
              tunnel: [w425 w442] -> w413
              tunnel: w414 -> [w429 w445]
              frame 1, Default {
                n162 = Unbundle By Name(w429) -> ("Wait Notifier"=w428:refnum<notifier>, "wait for reply"=w427:bool)
                n163 = local read "CAN_OBJ_RN"() -> (w433:T1[])
                n164 = dll-call lib="PTH2labs CUsers\n终极BOSS\tDocumentsCEPSLV300-1老性能试验台\tLibrariesZLG_CANControlCAN.dll" fn="VCI_Receive"(error in=w431, "DeviceType"=w436, "DeviceInd"=w435, "CANInd"=w434, "pReceive"=w433, "Len"=w430, "WaitTime"=100) -> (error out=w425:errorcluster, "pReceive"=w426:T1[])  [unwired: 7 in, 2 out]
                n165 = case shown="真" w427 {
                  tunnel: w428 -> [_ w441]
                  tunnel: w426 -> [_ w438]
                  tunnel: w425 -> [_ w437]
                  frame False {
                  }
                  frame True {
                    n166 = Bundle By Name(cluster=T21 {"Can_Receive"=[], "Recive_Wait_error"={"status"=FALSE, "code"=0, "source"=""}} ("Recive_Wait (Reply Payload)"), "Can_Receive"=w438, "Recive_Wait_error"=w437) -> (w439:T21)
                    n167 = Send Notification(notification=w439, notifier=w441) -> ()  [unwired: 1 in, 2 out]
                  }
                }
              }
              frame 0 {
                n168 = Unbundle By Name(w445) -> ("Wait Notifier"=w444:refnum<notifier>, "wait for reply"=w443:bool)
                n169 = case shown="真" w443 {
                  tunnel: w444 -> [_ w449]
                  tunnel: w442 -> [_ w446]
                  frame False {
                  }
                  frame True {
                    n170 = Bundle By Name(cluster=T21 {"Can_Receive"=[], "Recive_Wait_error"={"status"=FALSE, "code"=0, "source"=""}} ("Recive_Wait (Reply Payload)"), "Recive_Wait_error"=w446) -> (w447:T21)
                    n171 = Send Notification(notification=w447, notifier=w449) -> ()  [unwired: 1 in, 2 out]
                  }
                }
              }
            }
            n172 = Merge Errors(w415, w413) -> (w412:errorcluster)
          }
          frame "Sent_Recive" {
            w461 = u8 0 ("CAN_Bit_7")
            w462 = u8 0 items=["正常发送", "单次发送", "自发自收", "单次自发自收"] ("发送类型")
            n173 = Variant To Data(error in=w487, type=T15 {"ID"=0, "帧类型"=0, "帧格式"=0, "CAN_FRAME"={"[0]"=0, "[1]"=0, "[2]"=0, "[3]"=0, "[4]"=0, "[5]"=0, "[6]"=0, "[7]"=0}, "帧长度"=0, "Wait Notifier"=refnum, "wait for reply"=FALSE} ("Sent_Recive Argument"), Variant=w485) -> (data=w483:T15, error out=w455:errorcluster)
            n174 = Unbundle By Name(w483) -> ("Wait Notifier"=w454:refnum<notifier>, "wait for reply"=w453:bool, "ID"=w459:u32, "帧类型"=w452:u8, "帧格式"=w458:u8, "帧长度"=w457:u8, "CAN_FRAME"=w456:T10)
            n175 = local read "设备类型"() -> (w479:u32)
            n176 = local read "索引"() -> (w480:u32)
            n177 = local read "CAN 通道"() -> (w481:u32)
            n178 = To Unsigned Byte Integer(number=u32 0) -> (unsigned 8bit integer=w478:u8)
            n179 = Unbundle(w456) -> ("[0]"=w476:u8, "[1]"=w475:u8, "[2]"=w474:u8, "[3]"=w473:u8, "[4]"=w472:u8, "[5]"=w471:u8, "[6]"=w470:u8, "[7]"=w469:u8)
            n180 = Bundle(cluster=T19 {"ID"=0, "TimeStamp"=0, "TimeFlag"=0, "SendType"=0, "RemoteFlag"=0, "ExternFlag"=0, "DataLen"=0, "CAN_Bit_0"=0, "CAN_Bit_1"=0, "CAN_Bit_2"=0, "CAN_Bit_3"=0, "CAN_Bit_4"=0, "CAN_Bit_5"=0, "CAN_Bit_6"=0, "CAN_Bit_7"=0, "CAN_Bit_8"=0, "CAN_Bit_9"=0, "CAN_Bit_10"=0} ("VCI_CAN_OBJ_T"), "ID"=w459, "TimeStamp"=u32 0, "TimeFlag"=w478, "SendType"=w462, "RemoteFlag"=w452, "ExternFlag"=w458, "DataLen"=w457, "CAN_Bit_0"=w476, "CAN_Bit_1"=w475, "CAN_Bit_2"=w474, "CAN_Bit_3"=w473, "CAN_Bit_4"=w472, "CAN_Bit_5"=w471, "CAN_Bit_6"=w470, "CAN_Bit_7"=w469, "CAN_Bit_8"=w461, "CAN_Bit_9"=w461, "CAN_Bit_10"=w461) -> (w477:T19)
            n181 = dll-call lib="PTH2labs CUsers\n终极BOSS\tDocumentsCEPSLV300-1老性能试验台\tLibrariesZLG_CANControlCAN.dll" fn="VCI_Transmit"(error in=w455, "DeviceType"=w479, "DeviceInd"=w480, "CANInd"=w481, "pSend"=w477, "Len"=u32 1) -> (error out=w467:errorcluster, "return type"=w468:u32, "pSend"=w466:T19)  [unwired: 6 in, 1 out]
            n182 = case shown="1" w468 {
              tunnel: w467 -> [w488 w491]
              tunnel: w466 -> [_ _]
              tunnel: w479 -> [_ w496]
              tunnel: w480 -> [_ w495]
              tunnel: w481 -> [_ w494]
              tunnel: [w488 w490] -> w450
              tunnel: [_ w489] -> w451
              frame 0, Default {
              }
              frame 1 {
                n183 = dll-call lib="PTH2labs CUsers\n终极BOSS\tDocumentsCEPSLV300-1老性能试验台\tLibrariesZLG_CANControlCAN.dll" fn="VCI_GetReceiveNum"(error in=w491, "DeviceType"=w496, "DeviceInd"=w495, "CANInd"=w494) -> (error out=w492:errorcluster, "return type"=w493:u32)  [unwired: 5 in, 1 out]
                n184 = case shown="1, 默认" w493 {
                  selector: w493 -> [_ w501]
                  tunnel: w496 -> [_ w504]
                  tunnel: w495 -> [_ w503]
                  tunnel: w494 -> [_ w502]
                  tunnel: [_ w500] -> w489
                  tunnel: w492 -> [w497 w499]
                  tunnel: [w497 w498] -> w490
                  frame 0 {
                  }
                  frame 1, Default {
                    n185 = local read "CAN_OBJ_RN"() -> (w506:T1[])
                    n186 = dll-call lib="PTH2labs CUsers\n终极BOSS\tDocumentsCEPSLV300-1老性能试验台\tLibrariesZLG_CANControlCAN.dll" fn="VCI_Receive"(error in=w499, "DeviceType"=w504, "DeviceInd"=w503, "CANInd"=w502, "pReceive"=w506, "Len"=w501, "WaitTime"=100) -> (error out=w498:errorcluster, "pReceive"=w500:T1[])  [unwired: 7 in, 2 out]
                  }
                }
              }
            }
            n187 = case shown="真" w453 {
              tunnel: w454 -> [_ w511]
              tunnel: w451 -> [_ w508]
              tunnel: w450 -> [_ w507]
              frame False {
              }
              frame True {
                n188 = Bundle By Name(cluster=T22 {"Receive"=[], "Sent_Recive_error"={"status"=FALSE, "code"=0, "source"=""}} ("Sent_Recive (Reply Payload)"), "Receive"=w508, "Sent_Recive_error"=w507) -> (w510:T22)
                n189 = Send Notification(notification=w510, notifier=w511) -> ()  [unwired: 1 in, 2 out]
              }
            }
            n190 = Merge Errors(w455, w450) -> (w482:errorcluster)
          }
          frame "---Copy This Frame---" {
            # "Duplicate this frame when creating new messages.  Change this comment in the duplicated frame to describe this message."
            n191 = Merge Errors(w514) -> (w513:errorcluster)
          }
          frame "--- Exit and Error Handling---" {
            # "Separator - The following cases handle errors and exit messages."
          }
          frame "Simulate MHL Error" {
            # "Simulate an error occurring at the MHL"
            n192 = call "Module Name--constant.vi"() -> ("Module Name"=w517:string)  [unwired: 11 in]
            n193 = xnode "Error Ring"("参数 0"=w517) -> ("错误输出"=w519:errorcluster)
            n194 = Merge Errors(w521, w519) -> (w520:errorcluster)
          }
          frame "Error" {
            # "Error - Check the error message data and respond accordingly. This message is sent by the \"Error Handler\" VIs at the end of each loop in this application."
            n195 = property class="Module Admin"(reference=w530) -> ("Accessors:External Launch"=w529:bool)  [unwired: 1 in, 2 out]
            n196 = Variant To Data(error in=w538, type=errorcluster {"status"=FALSE, "code"=0, "source"=""} ("error constant"), Variant=w532) -> (data=w539:errorcluster, error out=w536:errorcluster)
            n197 = call "Error Reported.vi"("Error"=w539) -> ()  [unwired: 10 in, 1 out]
            n198 = case shown="假" w529 {
              tunnel: [w544 _] -> w535
              tunnel: w531 -> [w542 _]
              tunnel: w539 -> [w543 _]
              frame False {
                n199 = call <vilib>:"Simple Error Handler.vi"("error in (no error)"=w543) -> ()  [unwired: 4 in, 5 out]
                n200 = call-poly <vilib>:"Delacor_lib_QMH_Enqueue Message (poly).vi"("Priority Message? (F)"=TRUE, "Message"="Exit", "Message Queue in"=w542) -> ("error out"=w544:errorcluster)  [unwired: 7 in, 1 out]
              }
              frame True {
                # "If the module was launched externally, calling the Error Reported broadcast VI is the only action performed by the \"Error\" message. The module's caller can then process the error appropriately."
              }
            }
            n201 = Merge Errors(w536, w535) -> (w534:errorcluster)
            n202 = local write "error out"(w534) -> ()
          }
          frame "Exit" {
            w549 = 91  # 91: not all Exit messages will have an argument
            w551 = TRUE  # Stop the VI
            # "Exit - Exit the application."
            n203 = Variant To Data(error in=w559, type=T5 {"Origin"="", "Exit via Stop Module Req?"=FALSE, "Wait for Module to stop?"=FALSE} ("Stop Argument"), Variant=w550) -> (data=w547:T5, error out=w555:errorcluster)
            n204 = call <vilib>:"Clear Errors.vi"("error in (no error)"=w555, "specific error code to clear (0: all)"=w549) -> ("error out"=w558:errorcluster)  [unwired: 4 in, 1 out]
            n205 = control-ref of="This VI"() -> (w546:refnum<vi>)
            n206 = call-dynamic "Delacor_lib_QMH_Release Message Queue.vi"("error in"=w558, "Message Queue"=w553) -> ("error out"=w557:errorcluster)  [unwired: 9 in]
            n207 = call "Handle Exit.vi"("Stop Argument"=w547, "Admin in"=w545, "VI reference"=w546) -> ("error out"=w554:errorcluster)  [unwired: 7 in, 1 out]
            n208 = Merge Errors(w557, w554) -> (w556:errorcluster)
          }
          frame Default {
            # "'Default' case only runs if there is a message that isn't defined in any of the other cases.  Output a programming error."
            n209 = call "Module Name--constant.vi"() -> ("Module Name"=w560:string)  [unwired: 11 in]
            n210 = xnode "Error Ring"("参数 0"=w561, "参数 1"=w560) -> ("错误输出"=w565:errorcluster)
            n211 = Merge Errors(w563, w565) -> (w564:errorcluster)
          }
        }
        n212 = call-dynamic "Delacor_lib_QMH_Error Handler - Message Handling Loop.vi"("error in"=w170, "Message Queue in"=w160) -> ("dup error in"=w167:errorcluster)  [unwired: 8 in, 1 out]
      }
    }
    frame Error {
      # "Synchronize Caller Events.vi will inform Start Module.vi that the module has launched and will let the code calling Start Module.vi register for broadcasts and would permit the caller receive the broadcast that an error occurred at launch time."
      n213 = call "Synchronize Caller Events.vi"("Singleton Module Admin in"=w574) -> ("error out"=w579:errorcluster)  [unwired: 9 in, 1 out]
      n214 = call "Module Name--constant.vi"() -> ("Module Name"=w577:string)  [unwired: 11 in]
      n215 = Format Into String(format string="An error occurred during initialization. %s is no longer running.", w577) -> (resulting string=w575:string)  [unwired: 2 in, 1 out]
      n216 = Merge Errors(w581, w579) -> (w580:errorcluster)
      n217 = call "Error Reported.vi"("Additional Information"=w575, "Error"=w580) -> ()  [unwired: 9 in, 1 out]
    }
  }
  n218 = Merge Errors(w14, w17) -> (w13:errorcluster)
  n219 = call "Close Module.vi"("error in (no error)"=w13, "Module Admin in"=w8) -> ("error out"=w15:errorcluster, "External Launch"=w1:bool, "Module Admin out"=w2:refnum<class "Delacor_lib_QMH_Module Admin.lvclass">)  [unwired: 7 in]
  n220 = Unregister For Events(event registration refnum=w7, error in=w15) -> (error out=w12:errorcluster)
  "error out" <- w12
  n221 = local write "Module Admin"(w2) -> ()
  n222 = case "External Launch?" shown="真" w1 {
    tunnel: w12 -> [_ w582]
    frame False {
    }
    frame True {
      n223 = case "条件结构" shown="无错误" w582 {
        frame No Error {
          n224 = invoke class="VI" method="FP.Close"() -> ()  [unwired: 3 in, 3 out]
        }
        frame Error {
          n225 = invoke class="VI" method="FP.Open"("Activate"=TRUE ("Activate?")) -> ()  [unwired: 4 in, 5 out]
        }
      }
    }
  }
